vi "FGV_ApplicationConfig.vi"(7 "Command":T3, 8 "error in (no error)":errorcluster, 11 "ApplicationConfigIn":T1) -> (0 "error out":errorcluster, 3 "ApplicationConfigOut":T1)   [LabVIEW 2013]
uses:
  Ctrls/EnumFgvConfigCommand.ctl
  Ctrls/ApplicationConfig.ctl
  Ctrls/MessageHandlerConfig.ctl
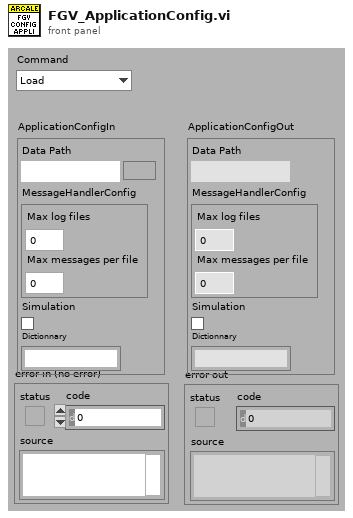
[diagram p1: front panel]
types:
  T1 = typedef "ApplicationConfig.ctl" = cluster{"Data Path":path, "MessageHandlerConfig":T2, "Simulation":bool, "Dictionnary":string}
  T2 = typedef "MessageHandlerConfig.ctl" = cluster{"Max log files":u32, "Max messages per file":u32}
  T3 = typedef "EnumFgvConfigCommand.ctl" = enum16{"Load", "Get", "Set", "Save To Disk"}
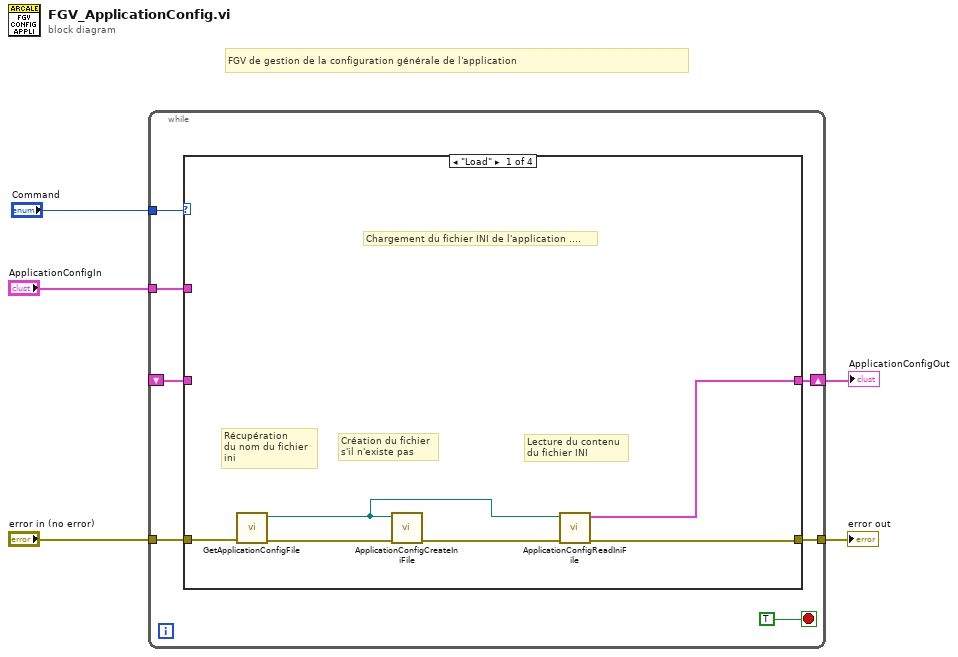
[diagram p0: block diagram]
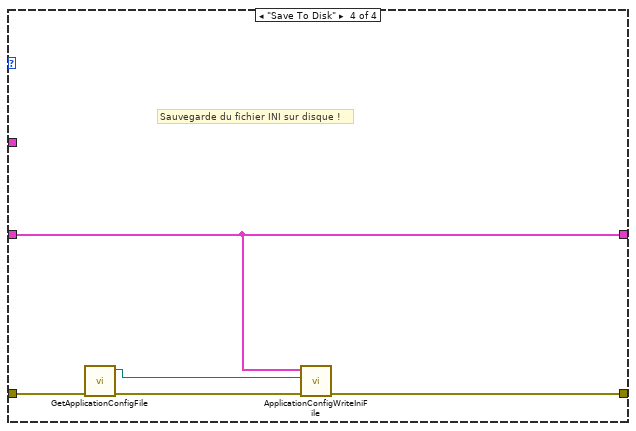
[diagram p4: hidden frame]
diagram:
  # "FGV de gestion de la configuration générale de l'application"
  n1 = while {
    tunnel: "Command" -> [w11]
    tunnel: "error in (no error)" -> [w10]
    tunnel: "ApplicationConfigIn" -> [w9]
    shift-right: [w8] -> w2
    shift-left: _ -> [w7]
    tunnel: [w6] -> w1
    stop <- TRUE stop-if-true
    n2 = case shown="\"Load\"" w11 {
      tunnel: w10 -> [w18 w19 w21 w26]
      tunnel: w9 -> [_ _ w22 _]
      tunnel: [w13 w20 w22 w23] -> w8
      tunnel: w7 -> [_ w20 _ w23]
      tunnel: [w16 w19 w21 w27] -> w6
      frame "Load" {
        # "Chargement du fichier INI de l'application ...."
        # "Lecture du contenu\ndu fichier INI"
        # "Création du fichier\ns'il n'existe pas"
        # "Récupération \ndu nom du fichier\nini"
        n3 = call "GetApplicationConfigFile.vi"("error in (no error)"=w18) -> ("error out"=w17:errorcluster, "Application config file Path"=w14:path)  [unwired: 9 in]
        n4 = call "ApplicationConfigCreateIniFile.vi"("error in (no error)"=w17, "Nom Fichier ini"=w14) -> ("error out"=w15:errorcluster)  [unwired: 9 in]
        n5 = call "ApplicationConfigReadIniFile.vi"("error in (no error)"=w15, "IniFilePath"=w14) -> ("error out"=w16:errorcluster, "ApplicationConfig"=w13:T1)  [unwired: 8 in]
      }
      frame "Get" {
      }
      frame "Set" {
      }
      frame "Save To Disk" {
        # "Sauvegarde du fichier INI sur disque !"
        n6 = call "GetApplicationConfigFile.vi"("error in (no error)"=w26) -> ("error out"=w25:errorcluster, "Application config file Path"=w24:path)  [unwired: 9 in]
        n7 = call "ApplicationConfigWriteIniFile.vi"("error in (no error)"=w25, "IniFilePath"=w24, "ApplicationConfig"=w23) -> ("error out"=w27:errorcluster)  [unwired: 8 in]
      }
    }
  }
  "error out" <- w1
  "ApplicationConfigOut" <- w2
